vi "init_LCD(SubVI).vi"   [LabVIEW 2015]
uses:
  <vilib>/myRIO/Instrument Drivers/Onboard IO/PWM/typedefs/PWM Reference.ctl
  <vilib>/myRIO/Common/Instrument Driver Framework/Utilities/typedefs/myRIO Generic Hardware Reference.ctl
  <vilib>/myRIO/Common/Instrument Driver Framework/Utilities/typedefs/Hardware Version Enum.ctl
  <vilib>/myRIO/Common/Instrument Driver Framework/Utilities/typedefs/myRIO v1.0 Reference.ctl
  <vilib>/myRIO/Common/Instrument Driver Framework/Utilities/typedefs/Generic FPGA Reference.ctl
  <vilib>/myRIO/Common/Instrument Driver Framework/myRIO v1.0/PWM/typedefs/PWM Channels Enum.ctl
  <vilib>/myRIO/Instrument Drivers/Onboard IO/PWM/typedefs/PWM Configuration.ctl
  <vilib>/userdefined/High Color/nirio_resource_hc.ctl
  <vilib>/myRIO/Instrument Drivers/Onboard IO/DIO/typedefs/DIO Reference.ctl
  <vilib>/myRIO/Common/Instrument Driver Framework/myRIO v1.0/DIO/typedefs/DIO Channels List.ctl
  <vilib>/myRIO/Common/Instrument Driver Framework/myRIO v1.0/DIO/typedefs/DIO Channels Enum.ctl
  <vilib>/myRIO/Common/Instrument Driver Framework/Utilities/vis/Is FPGA Ref Available.vi
  <vilib>/myRIO/Common/Instrument Driver Framework/myRIO v1.0/PWM/vis/myRIO v1.1 Open PWM.vi
  <vilib>/myRIO/Instrument Drivers/Onboard IO/PWM/vis/Set Duty Cycle and Frequency.vi
  <vilib>/myRIO/Common/Instrument Driver Framework/myRIO v1.0/DIO/vis/myRIO v1.1 Open DIO.vi
  <vilib>/myRIO/Instrument Drivers/Onboard IO/DIO/vis/Write.vi
  <vilib>/myRIO/Common/Instrument Driver Framework/Utilities/vis/Validate Channels.vi
  <vilib>/myRIO/Common/Instrument Driver Framework/myRIO v1.0/PWM/vis/myRIO v1.0 Reserve PWM.vi
  <vilib>/myRIO/Common/Instrument Driver Framework/myRIO v1.0/DIO/vis/myRIO v1.0 Reserve DIO.vi
  <vilib>/myRIO/Common/Instrument Driver Framework/myRIO v1.0/PWM/vis/myRIO v1.0 Build MUX Configuration PWM.vi
  <vilib>/myRIO/Common/Instrument Driver Framework/myRIO v1.0/Resource Manager/vis/myRIO v1.0 Reserve Channel List.vi
  <vilib>/myRIO/Common/Instrument Driver Framework/myRIO v1.0/DIO/vis/myRIO v1.0 Build MUX Configuration DIO.vi
  <vilib>/myRIO/Common/Instrument Driver Framework/myRIO v1.0/Resource Manager/vis/myRIO v1.0 Create Configuration List.vi
  <vilib>/myRIO/Common/Instrument Driver Framework/myRIO v1.0/Resource Manager/vis/myRIO v1.0 Reserve Channel.vi
  <vilib>/myRIO/Common/Instrument Driver Framework/myRIO v1.0/Resource Manager/vis/myRIO v1.0 Unreserve Channel.vi
  <vilib>/myRIO/Common/Instrument Driver Framework/myRIO v1.0/Resource Manager/vis/myRIO v1.0 Build Mutex Name.vi
  <vilib>/Utility/VariantDataType/GetNumericInfo.vi
  <vilib>/Utility/error.llb/Error Cluster From Error Code.vi
  <vilib>/myRIO/Common/Instrument Driver Framework/myRIO v1.0/myRIO v1.1 Open.vi
  <vilib>/myRIO/Common/Instrument Driver Framework/Utilities/vis/IO Manager.vi
  <vilib>/myRIO/Common/Instrument Driver Framework/Utilities/vis/Configuration Manager.vi
  <vilib>/myRIO/Common/Instrument Driver Framework/myRIO v1.0/Resource Manager/vis/myRIO v1.0 Configure IO.vi
  <vilib>/myRIO/Common/Instrument Driver Framework/myRIO v1.0/myRIO v1.0 Close.vi
  <vilib>/myRIO/Common/Instrument Driver Framework/myRIO v1.0/DIO/vis/myRIO v1.0 Write DIO.vi
  <vilib>/myRIO/Common/Instrument Driver Framework/myRIO v1.0/PWM/vis/myRIO v1.0 Write PWM.vi
  <vilib>/myRIO/Express VI/Onboard IO/DO/DO Express VI.xnode
  <vilib>/myRIO/Instrument Drivers/Onboard IO/DIO/vis/myRIO DIO Open.xnode
  <vilib>/myRIO/Express VI/Onboard IO/PWM/PWM Express VI.xnode
  <vilib>/myRIO/Instrument Drivers/Onboard IO/PWM/vis/myRIO PWM Open.xnode
  <vilib>/myRIO/Instrument Drivers/Onboard IO/DIO/DIO.lvlib
  <vilib>/myRIO/Instrument Drivers/Onboard IO/PWM/PWM.lvlib
types:
  T1 = typedef "DIO.lvlib/DIO Reference.ctl" = cluster{"myRIO Reference":T2, "DIO Channels List":T6}
  T2 = typedef "myRIO Generic Hardware Reference.ctl" = cluster{"myRIO Model":T3, "myRIO Hardware Reference":T4}
  T3 = typedef "Hardware Version Enum.ctl" = enum16{"Unknown", "myRIO-1900", "myRIO-1950", "roboRIO"}
  T4 = typedef "myRIO v1.0 Reference.ctl" = cluster{"Generic FPGA Reference":T5, "Allow multiple opens":bool}
  T5 = typedef "Generic FPGA Reference.ctl" = refnum<k20>
  T6 = typedef "DIO Channels List.ctl" = T7[]
  T7 = typedef "DIO Channels Enum.ctl" = enum16{"Not Connected", "C/DIO0", "C/DIO1", "C/DIO2", "C/DIO3", "C/DIO4", "C/DIO5", "C/DIO6", "C/DIO7", "A/DIO0", "A/DIO1", "A/DIO2", "A/DIO3", "A/DIO4", "A/DIO5", "A/DIO6", "A/DIO7", "A/DIO8", "A/DIO9", "A/DIO10", "A/DIO11", "A/DIO12", "A/DIO13", "A/DIO14", "A/DIO15", "B/DIO0", "B/DIO1", "B/DIO2", "B/DIO3", "B/DIO4", "B/DIO5", "B/DIO6", "B/DIO7", "B/DIO8", "B/DIO9", "B/DIO10", "B/DIO11", "B/DIO12", "B/DIO13", "B/DIO14", "B/DIO15", "LED0", "LED1", "LED2", "LED3", "Button0", "DIO/DIO0", "DIO/DIO1", "DIO/DIO2", "DIO/DIO3", "DIO/DIO4", "DIO/DIO5", "DIO/DIO6", "DIO/DIO7", "DIO/DIO8", "DIO/DIO9", "SPI/CS0", "SPI/CS1", "SPI/CS2", "SPI/CS3", "LED RADIO (Green)", "LED RADIO (Red)", "LED COMM (Green)", "LED COMM (Red)", "LED MODE (Green)", "LED MODE (Red)"}
  T8 = typedef "nirio_resource_hc.ctl" = tag
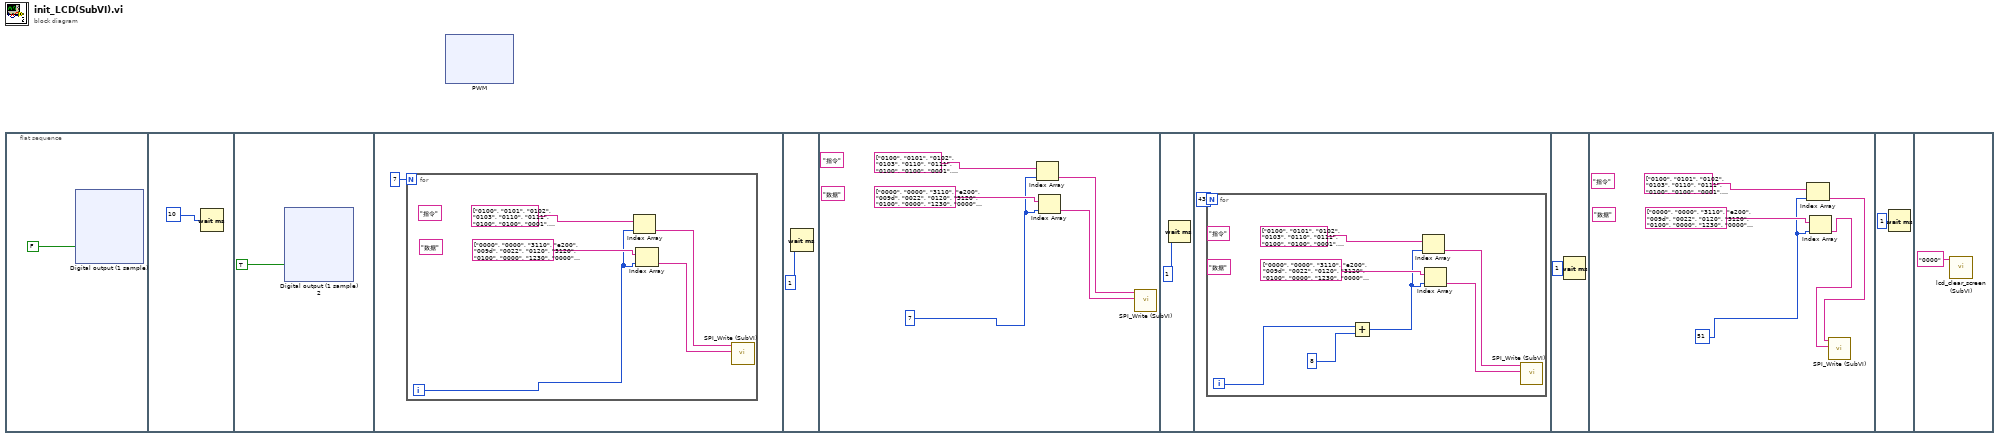
[diagram p0: block diagram]
diagram:
  n1 = flat-sequence {
    frame #0 {
      n2 = xnode "Digital output (1 sample)"("B/DIO2 (Pin 15)"=FALSE) -> ()  [unwired: 1 in, 1 out]
    }
    frame #1 {
      n3 = Wait (ms)(milliseconds to wait=u32 10) -> ()  [unwired: 1 out]
    }
    frame #2 {
      n4 = xnode "Digital output (1 sample) 2"("B/DIO2 (Pin 15)"=TRUE) -> ()  [unwired: 1 in, 1 out]
    }
    frame #3 {
      n5 = for {
        N: 7 -> [_]
        i -> [w75]
        (unwired) "数据"
        (unwired) "指令"
        n6 = Index Array(array=string[] ["0100", "0101", "0102", "0103", "0110", "0111", "0100", "0100", "0001", "0002", "0003", "0006", "0007", "0008", "0009", "000b", "000c", "000d", "0012", "0013", "0018", "0019", "0203", "0204", "0210", "0211", "0212", "0213", "0214", "0215", "0216", "0217", "0300", "0301", "0302", "0303", "0304", "0305", "0306", "0307", "0308", "0309", "0400", "0401", "0402", "0403", "0404", "0200", "0201", "0100", "0007", "0007"], index=w75) -> (element=w79:string)
        n7 = Index Array(array=string[] ["0000", "0000", "3110", "e200", "009d", "0022", "0120", "3120", "0100", "0000", "1230", "0000", "0101", "0808", "0000", "0000", "0000", "0018", "0000", "0000", "0000", "0000", "0000", "0000", "0000", "00ef", "0000", "013f", "0000", "0000", "0000", "0000", "5343", "1021", "0003", "0011", "050a", "4342", "1100", "0003", "1201", "050a", "4027", "0000", "0000", "013f", "0000", "0000", "0000", "7120", "0103", "0113"], index=w75) -> (element=w78:string)
        n8 = call "SPI_Write (SubVI).vi"("data"=w78, "index"=w79) -> ()  [unwired: 10 in]
      }
    }
    frame #4 {
      n9 = Wait (ms)(milliseconds to wait=u32 1) -> ()  [unwired: 1 out]
    }
    frame #5 {
      w81 = 7
      (unwired) "数据"
      (unwired) "指令"
      n10 = Index Array(array=string[] ["0100", "0101", "0102", "0103", "0110", "0111", "0100", "0100", "0001", "0002", "0003", "0006", "0007", "0008", "0009", "000b", "000c", "000d", "0012", "0013", "0018", "0019", "0203", "0204", "0210", "0211", "0212", "0213", "0214", "0215", "0216", "0217", "0300", "0301", "0302", "0303", "0304", "0305", "0306", "0307", "0308", "0309", "0400", "0401", "0402", "0403", "0404", "0200", "0201", "0100", "0007", "0007"], index=w81) -> (element=w85:string)
      n11 = Index Array(array=string[] ["0000", "0000", "3110", "e200", "009d", "0022", "0120", "3120", "0100", "0000", "1230", "0000", "0101", "0808", "0000", "0000", "0000", "0018", "0000", "0000", "0000", "0000", "0000", "0000", "0000", "00ef", "0000", "013f", "0000", "0000", "0000", "0000", "5343", "1021", "0003", "0011", "050a", "4342", "1100", "0003", "1201", "050a", "4027", "0000", "0000", "013f", "0000", "0000", "0000", "7120", "0103", "0113"], index=w81) -> (element=w84:string)
      n12 = call "SPI_Write (SubVI).vi"("data"=w84, "index"=w85) -> ()  [unwired: 10 in]
    }
    frame #6 {
      n13 = Wait (ms)(milliseconds to wait=u32 1) -> ()  [unwired: 1 out]
    }
    frame #7 {
      n14 = for {
        N: 43 -> [_]
        i -> [w89]
        (unwired) "数据"
        (unwired) "指令"
        n15 = Add(x=w89, y=8) -> (x+y=w88:i32)
        n16 = Index Array(array=string[] ["0100", "0101", "0102", "0103", "0110", "0111", "0100", "0100", "0001", "0002", "0003", "0006", "0007", "0008", "0009", "000b", "000c", "000d", "0012", "0013", "0018", "0019", "0203", "0204", "0210", "0211", "0212", "0213", "0214", "0215", "0216", "0217", "0300", "0301", "0302", "0303", "0304", "0305", "0306", "0307", "0308", "0309", "0400", "0401", "0402", "0403", "0404", "0200", "0201", "0100", "0007", "0007"], index=w88) -> (element=w91:string)
        n17 = Index Array(array=string[] ["0000", "0000", "3110", "e200", "009d", "0022", "0120", "3120", "0100", "0000", "1230", "0000", "0101", "0808", "0000", "0000", "0000", "0018", "0000", "0000", "0000", "0000", "0000", "0000", "0000", "00ef", "0000", "013f", "0000", "0000", "0000", "0000", "5343", "1021", "0003", "0011", "050a", "4342", "1100", "0003", "1201", "050a", "4027", "0000", "0000", "013f", "0000", "0000", "0000", "7120", "0103", "0113"], index=w88) -> (element=w92:string)
        n18 = call "SPI_Write (SubVI).vi"("data"=w92, "index"=w91) -> ()  [unwired: 10 in]
      }
    }
    frame #8 {
      n19 = Wait (ms)(milliseconds to wait=u32 1) -> ()  [unwired: 1 out]
    }
    frame #9 {
      w96 = 51
      (unwired) "数据"
      (unwired) "指令"
      n20 = Index Array(array=string[] ["0100", "0101", "0102", "0103", "0110", "0111", "0100", "0100", "0001", "0002", "0003", "0006", "0007", "0008", "0009", "000b", "000c", "000d", "0012", "0013", "0018", "0019", "0203", "0204", "0210", "0211", "0212", "0213", "0214", "0215", "0216", "0217", "0300", "0301", "0302", "0303", "0304", "0305", "0306", "0307", "0308", "0309", "0400", "0401", "0402", "0403", "0404", "0200", "0201", "0100", "0007", "0007"], index=w96) -> (element=w98:string)
      n21 = Index Array(array=string[] ["0000", "0000", "3110", "e200", "009d", "0022", "0120", "3120", "0100", "0000", "1230", "0000", "0101", "0808", "0000", "0000", "0000", "0018", "0000", "0000", "0000", "0000", "0000", "0000", "0000", "00ef", "0000", "013f", "0000", "0000", "0000", "0000", "5343", "1021", "0003", "0011", "050a", "4342", "1100", "0003", "1201", "050a", "4027", "0000", "0000", "013f", "0000", "0000", "0000", "7120", "0103", "0113"], index=w96) -> (element=w97:string)
      n22 = call "SPI_Write (SubVI).vi"("data"=w97, "index"=w98) -> ()  [unwired: 10 in]
    }
    frame #10 {
      n23 = Wait (ms)(milliseconds to wait=u32 1) -> ()  [unwired: 1 out]
    }
    frame #11 {
      n24 = call "lcd_clear_screen (SubVI).vi"("color blackground"="0000") -> ()  [unwired: 11 in]
    }
  }
  n25 = xnode "PWM"() -> ()  [unwired: 1 in, 1 out]
